vi "Interpolation Test (control).vi"() -> ()   [LabVIEW 2014]
uses:
  <vilib>/FPGAPlugInAG/sbRIO-9636/niLvFpga_Open_sbRIO-9636.vi
  <vilib>/rvi/interface/common/dynamic/niFpgaDynamicAddResources.vi
  <vilib>/Utility/error.llb/Error Cluster From Error Code.vi
  <vilib>/rvi/errors/niLvFpgaAdjustHostInterfaceError.vi
  <vilib>/FPGAPlugInAG/Dynamic/niLvFpga_Abort_Dynamic.vi
  <vilib>/FPGAPlugInAG/Dynamic/niLvFpga_Close_Dynamic.vi
  <vilib>/rvi/interface/nirviOpenFPGA/nirviOpenFPGA.xnode
  FPGA Bitfiles/LaserDistanceSen_FPGATarget_DoubleFFTMesuram_oR0WZ1FCw3Y.lvbitx
  FPGA Target/Test VIs/Double FFT Mesurament (Max Bin detection - Control) test.vi
  <vilib>/rvi/interface/nirviReadWriteControl/nirviReadWriteControl.xnode
  <vilib>/rvi/interface/nirviMethod/nirviMethod.xnode
  <vilib>/rvi/interface/nirviCloseFPGA/nirviCloseFPGA.xnode
  NiFpgaLv.dll
  <vilib>/rvi/interface/Simulation/niFpgaSimulationCallBeginRW.vi
panel:
  in  "first bin":i32=255
  in  "last bin":i32=10
  in  "lower limit 2":u32(slide) scale=625.0..737.0
  in  "lower limit 1":u32(slide) scale=0.0..112.0
  in  "Interpolation Method":T1(ring)
  out "Interpolated Bin":dbl
  out "Next Amp":dbl format="%.2f"
  out "Prev Amp":dbl format="%.2f"
  out "Next Bin":i32
  out "Prev Bin":i32
  out "Max Amp":dbl format="%.2f"
  out "Max Bin":i32
  in  "stop":bool
  out "Detected Frequency (Hz)":dbl
  # "FFT Limit for Max Computation\n(values between 0 and 255)"
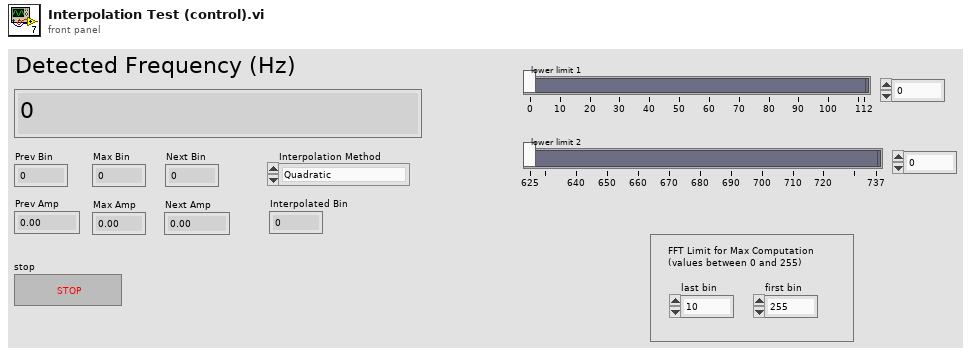
[diagram p1: front panel]
types:
  T1 = enum16{"Quadratic", "McLeodd", "Barycentric", "Jain"}
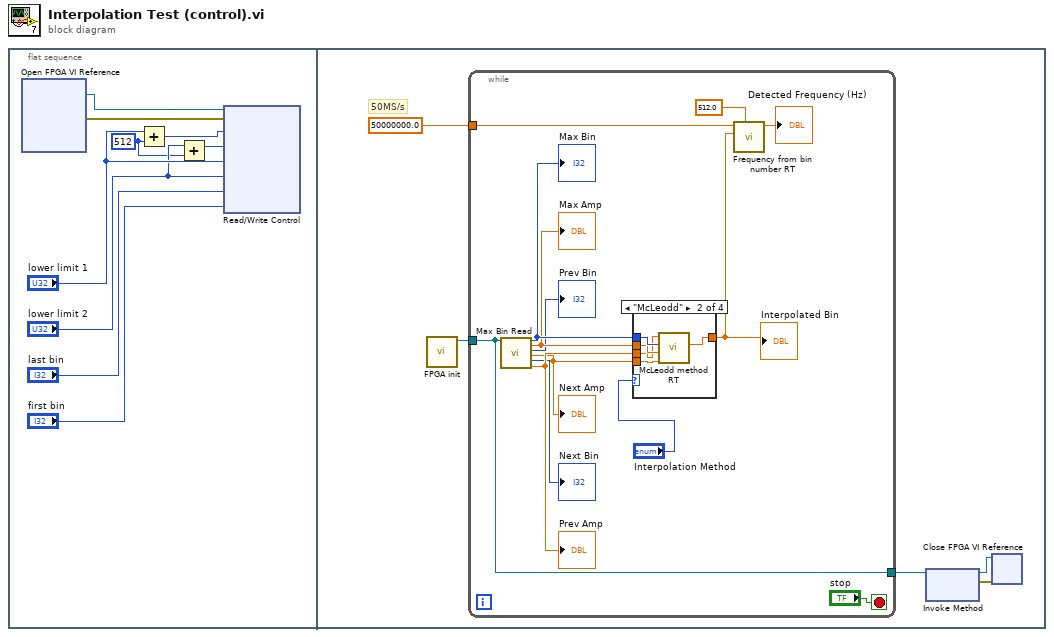
[diagram p0: block diagram]
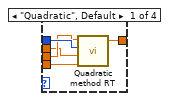
[diagram p2: hidden frame]
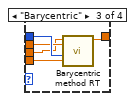
[diagram p3: hidden frame]
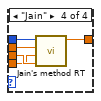
[diagram p4: hidden frame]
diagram:
  n1 = flat-sequence {
    frame #0 {
      w1 = u32 512 ("y")
      n2 = xnode "Open FPGA VI Reference"() -> ("FPGA VI Reference Out"=w9:refnum<k20>, "error out"=w8:errorcluster)  [unwired: 2 in]
      n3 = Add(x="lower limit 1", y=w1) -> (x+y=w5:u32)
      n4 = Add(x="lower limit 2", y=w1) -> (x+y=w3:u32)
      n5 = xnode "Read/Write Control"("FPGA VI Reference In"=w9, "error in"=w8, "upper limit 1"=w5, "upper limit 2"=w3, "lower limit 1"="lower limit 1", "lower limit 2"="lower limit 2", "last bin"="last bin", "first bin"="first bin") -> ()  [unwired: 2 out]
    }
    frame #1 {
      # "50MS/s"
      n6 = call "FPGA init.vi"() -> ("FPGA VI Reference Out"=w11:refnum<k20>)  [unwired: 10 in, 1 out]
      n7 = while {
        tunnel: w11 -> [w19]
        tunnel: 50000000.0 ("Sample Rate (S/s)") -> [w22]
        tunnel: [w19] -> w10
        stop <- "stop" stop-if-true
        n8 = call "Max Bin Read.vi"("FPGA VI Reference In"=w19) -> ("Max Bin"=w27:i32, "Max Amp"=w26:dbl, "Prev Bin"=→"Prev Bin":i32, "Next Amp"=w20:dbl, "Next Bin"=→"Next Bin":i32, "Prev Amp"=w21:dbl)  [unwired: 13 in]
        "Max Bin" <- w27
        "Max Amp" <- w26
        "Prev Amp" <- w21
        "Next Amp" <- w20
        n9 = case shown="\"McLeodd\"" "Interpolation Method" {
          tunnel: w27 -> [w31 w36 w41 w46]
          tunnel: w26 -> [w28 w35 w40 w45]
          tunnel: w21 -> [w29 w34 w39 w44]
          tunnel: w20 -> [w30 w33 w38 w43]
          tunnel: [w32 w37 w42 w47] -> w16
          frame "Quadratic", Default {
            n10 = call "Quadratic method RT.vi"("Next Amplitude"=w30, "Max Amplitude"=w28, "Max bin"=w31, "Prev Amplitude"=w29) -> ("Bin"=w32:dbl)  [unwired: 7 in]
          }
          frame "McLeodd" {
            n11 = call "McLeodd method RT.vi"("Next Amp"=w33, "Max Amp"=w35, "Max Bin"=w36, "Prev Amp"=w34) -> ("Bin"=w37:dbl)  [unwired: 7 in]
          }
          frame "Barycentric" {
            n12 = call "Barycentric method RT.vi"("Next Amp"=w38, "Max Bin"=w41, "Max Amp"=w40, "Prev Amp"=w39) -> ("Bin"=w42:dbl)  [unwired: 7 in]
          }
          frame "Jain" {
            n13 = call "Jain's method RT.vi"("Prev Amp"=w44, "Next Amp"=w43, "Max Amp"=w45, "Max Bin"=w46) -> ("Bin"=w47:dbl)  [unwired: 7 in]
          }
        }
        "Interpolated Bin" <- w16
        n14 = call "Frequency from bin number RT.vi"("FFT size"=512.0, "Bin number"=w16, "Sample Rate (S/s)"=w22) -> ("Detected Frequency (Hz)"=→"Detected Frequency (Hz)":dbl)  [unwired: 8 in]
      }
      n15 = xnode "Invoke Method"("FPGA VI Reference In"=w10) -> ("FPGA VI Reference Out"=w13:refnum<k20>, "error out"=w12:errorcluster)  [unwired: 1 in]
      n16 = xnode "Close FPGA VI Reference"("FPGA VI Reference In"=w13, "error in"=w12) -> ()  [unwired: 1 out]
    }
  }
